vi "ErrorHandling.getErrorsFromTo.vi"(0 "ErrorHandling in":refnum<class "ErrorHandling.lvclass">, 2 "TimestampFrom":timestamp, 3 "TimestampTo":timestamp, 5 "error in (no error)":errorcluster) -> (14 "ErrorHandling out":refnum<class "ErrorHandling.lvclass">, 16 "Errors":T1[](array[typedef]), 19 "error out":errorcluster)   [LabVIEW 2016, in "ErrorHandling.lvclass"]
doc: "Gibt die Fehler Von .. bis .. aus\n\n27.05.14 / sige"
uses:
  ErrorHandling.lvclass
  ErrorHandling.OccurredErrorDataStruct.ctl
  ErrorHandling.lvclass/ErrorHandling.ctl
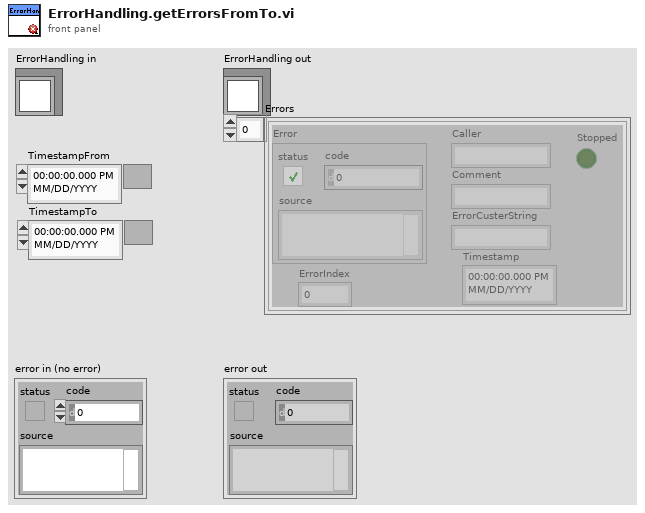
[diagram p1: front panel]
types:
  T1 = typedef "ErrorHandling.lvclass/ErrorHandling.OccurredErrorDataStruct.ctl" = cluster{"Error":errorcluster, "Caller":string, "Comment":string, "Timestamp":timestamp, "Stopped":bool, "ErrorCusterString":string, "ErrorIndex":u64}
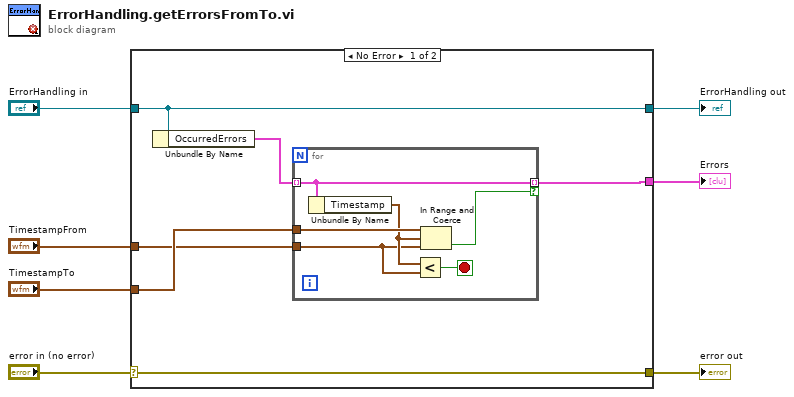
[diagram p0: block diagram]
diagram:
  n1 = case shown="No Error" "error in (no error)" {
    selector: "error in (no error)" -> [w13 w21]
    tunnel: [w13 w21] -> w6
    tunnel: [w12 w20] -> w4
    tunnel: "ErrorHandling in" -> [w12 w20]
    tunnel: [w8 _] -> w3
    tunnel: "TimestampFrom" -> [w9 _]
    tunnel: "TimestampTo" -> [w10 _]
    frame No Error {
      n2 = Unbundle By Name(w12) -> ("OccurredErrors"=w11:T1[])
      n3 = for {
        tunnel: w11 -> [w19] mode=indexing
        tunnel: [w19] -> w8 mode=indexing if=w17
        tunnel: w10 -> [w18]
        tunnel: w9 -> [w15]
        stop <- w14 stop-if-true
        n4 = Unbundle By Name(w19) -> ("Timestamp"=w16:timestamp)
        n5 = Less?(x=w16, y=w15) -> (x < y?=w14:bool)
        n6 = In Range and Coerce(upper limit=w18, x=w16, lower limit=w15) -> (In Range?=w17:bool)  [unwired: 1 out]
      }
    }
    frame Error {
    }
  }
  "error out" <- w6
  "ErrorHandling out" <- w4
  "Errors" <- w3
